vi "Write Data Types.vi"(4 "Data Type Handler":refnum<class "Test Executive Builder Data Type Handler.lvclass">, 6 "Data Type Views":refnum<class "IAttribute Data Type View.lvclass">[](array[class]), 11 "Test Executive Builder in":refnum<class "Test Executive Builder.lvclass">) -> (3 "Test Executive Builder out":refnum<class "Test Executive Builder.lvclass">)   [LabVIEW 2019, in "Test Executive Builder.lvclass"]
uses:
  <vilib>/gpm_packages/@cs/Test-executive-builder/Example/Application/Test Executive Builder/Test Executive Builder/Test Executive Builder.lvclass
  <vilib>/gpm_packages/@cs/Test-executive-builder/Source/Test Executive Builder Dialogs/IAttribute Data Type View/IAttribute Data Type View.lvclass
  <vilib>/gpm_packages/@cs/Test-executive-builder/Source/Data Type Handler/Test Executive Builder Data Type Handler.lvclass
  <vilib>/gpm_packages/@cs/Test-executive-builder/Example/Application/Test Executive Builder/Test Executive Builder/Test Executive Builder.lvclass/Test Executive Builder.ctl
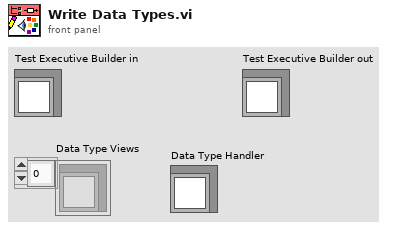
[diagram p1: front panel]
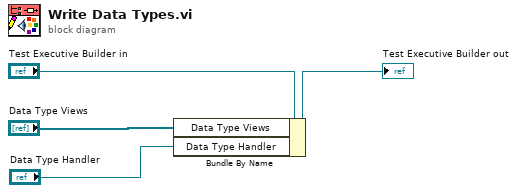
[diagram p0: block diagram]
diagram:
  n1 = Bundle By Name(cluster="Test Executive Builder in", "Data Type Views"="Data Type Views", "Data Type Handler"="Data Type Handler") -> (→"Test Executive Builder out":refnum<class "Test Executive Builder.lvclass">)
